vi "FL_map MAX single side.vi"(7 "X(Max)":dbl, 9 "x_l":dbl, 11 "x_r":dbl, 12 "x0":dbl, 13 "x1":dbl, 14 "x2":dbl, 15 "x3":dbl) -> (8 "X(Max)":dbl)   [LabVIEW 2013, in "NI_Fuzzy_Logic_API.lvlib"]
uses:
  <vilib>/addons/Fuzzy Logic/NI_Fuzzy_Logic_API.lvlib
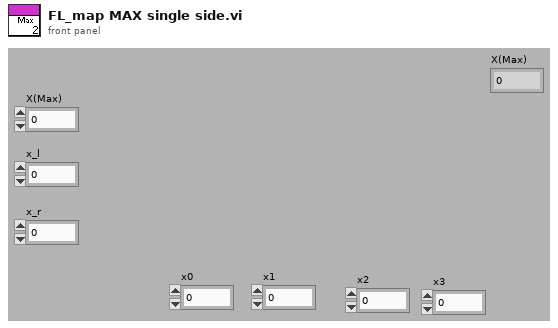
[diagram p1: front panel]
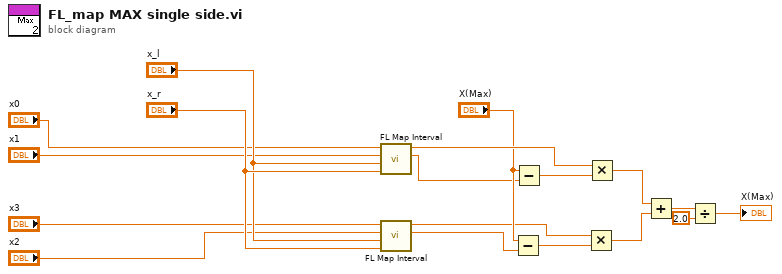
[diagram p0: block diagram]
diagram:
  n1 = call <vilib>:"FL Map Interval.vi"("x1"="x_r", "x0"="x_l", "b"="x1", "a"="x0") -> ("m"=w16:dbl, "k"=w18:dbl)  [unwired: 6 out]
  n2 = call <vilib>:"FL Map Interval.vi"("x1"="x_r", "x0"="x_l", "b"="x2", "a"="x3") -> ("m"=w11:dbl, "k"=w12:dbl)  [unwired: 6 out]
  n3 = Subtract(x="X(Max)", y=w11) -> (x-y=w10:dbl)
  n4 = Subtract(x="X(Max)", y=w16) -> (x-y=w15:dbl)
  n5 = Multiply(x=w12, y=w10) -> (x*y=w3:dbl)
  n6 = Multiply(x=w18, y=w15) -> (x*y=w2:dbl)
  n7 = Add(x=w2, y=w3) -> (x+y=w8:dbl)
  n8 = Divide(x=w8, y=2.0) -> (x/y=→"X(Max)":dbl)
